vi "Validate message.vi"(0 "multipart message in":string[](array[string]), 11 "error in (no error)":errorcluster) -> (3 "Command Type":T1=enum."instrument_control", 4 "multipart message out":string[](array[string]), 6 "command out":T2=enum."configure_rf", 10 "Valid message?":bool, 14 "Debug info":string, 15 "error out":errorcluster)   [LabVIEW 2019, in "mmW_commands.lvlib"]
doc: "- Validate received message\no check if ZMQ multipart message has (exactly) 3 string elements -> PASS/FAIL\no IF PASSED:\n\" …\n\" extract command > enum\n\" decide if it's instrument command or environment control command type"
uses:
  mmW_commands.lvlib
  TypeDefs/commands.ctl
  TypeDefs/command_types.ctl
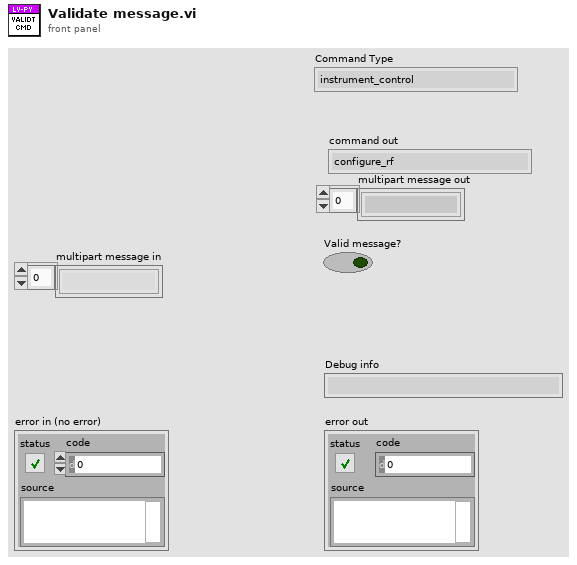
[diagram p1: front panel]
types:
  T1 = typedef "mmW_commands.lvlib/command_types.ctl" = enum16{"invalid_command", "instrument_control", "environment_control", "response"}
  T2 = typedef "mmW_commands.lvlib/commands.ctl" = enum16{"configure_fs", "configure_rf", "configure_trigger", "equalization_enable", "equalization_start", "lo_sync_enable", "equalization_stop", "get_instrument_status", "get_versions", "initialize_hw", "pop_rx", "set_log_level", "Shutdown", "start", "start_instrument_app", "stop", "trans", "transceive", "trigger_burst", "trigger_sync_enable", "Write TX", "resp_generic", "resp_waveform", "send_trigger", "fetch", "transceive2"}
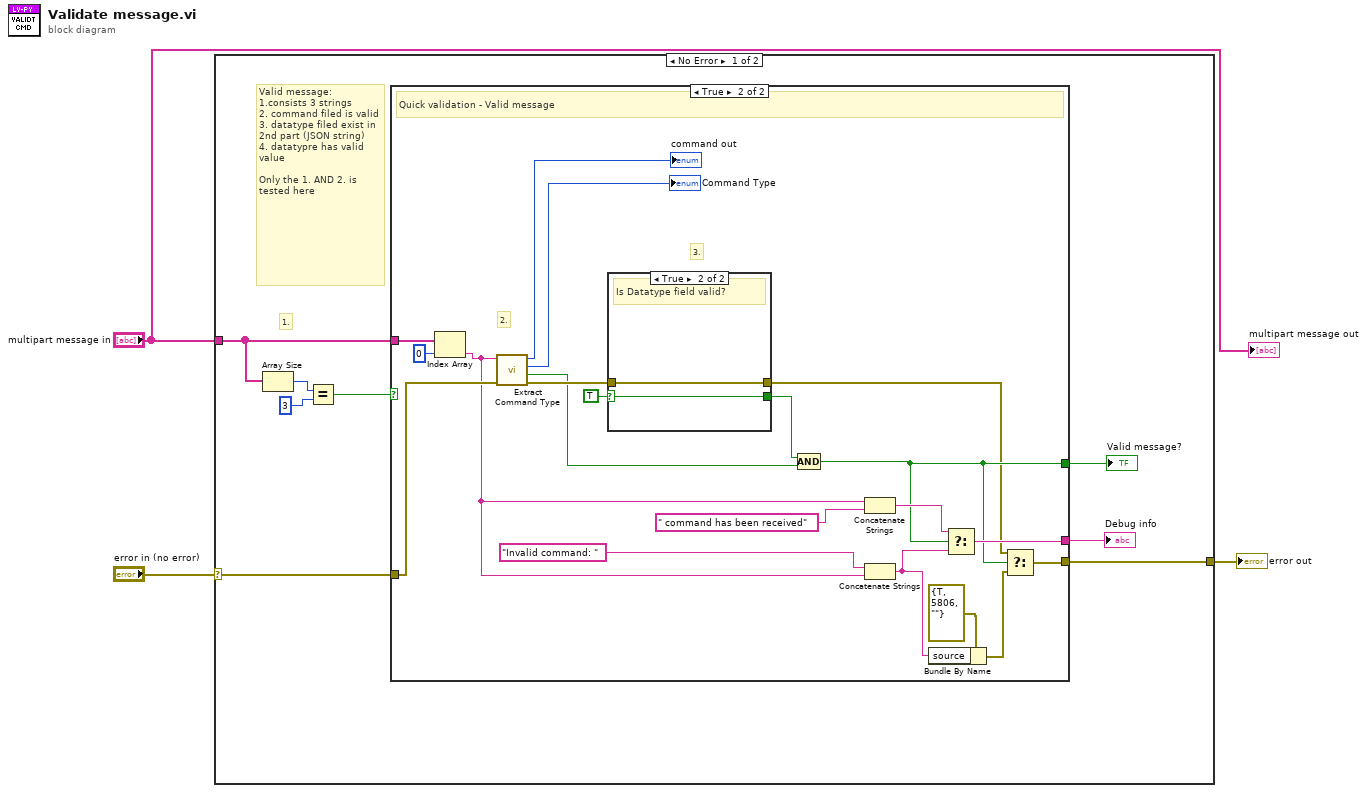
[diagram p0: block diagram]
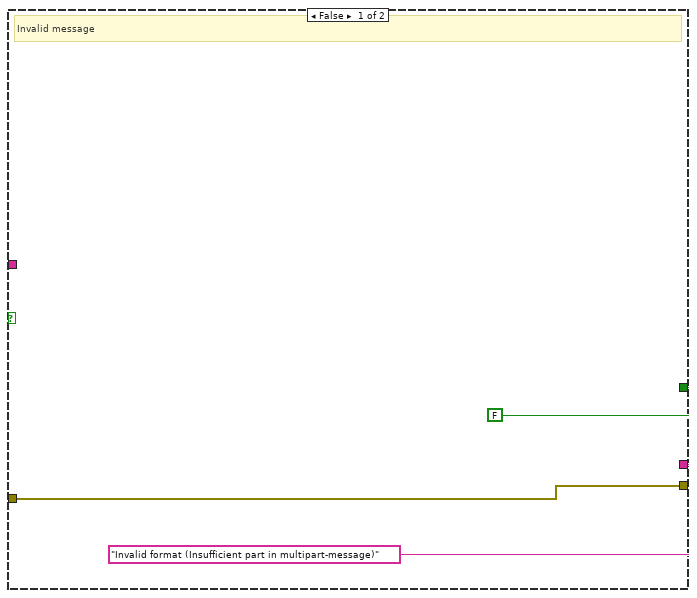
[diagram p2: hidden frame]
diagram:
  n1 = case shown="No Error" "error in (no error)" {
    selector: "error in (no error)" -> [w4 w39]
    tunnel: "multipart message in" -> [w10 _]
    tunnel: [w5 w39] -> w2
    frame No Error {
      # "1."
      # "Valid message:\n1.consists 3 strings\n2. command filed is valid\n3. datatype filed exist in 2nd part (JSON string)\n4. datatypre has valid value\n\nOnly the 1. AND 2. is tested here"
      n2 = Array Size(array=w10) -> (size(s)=w7:i32)
      n3 = Equal?(x=w7, y=3) -> (x = y?=w9:bool)
      n4 = case shown="True" w9 {
        tunnel: w4 -> [w13 w30]
        tunnel: w10 -> [_ w25]
        tunnel: [FALSE w17] -> w6
        tunnel: [w13 w29] -> w5
        tunnel: ["Invalid format (Insufficient part in multipart-message)" w32] -> w11
        frame False {
          # "Invalid message"
        }
        frame True {
          # "3."
          # "2."
          # "Quick validation - Valid message"
          n5 = Index Array(array=w25, index=0) -> (element=w16:string)
          n6 = call "Extract Command Type.vi"("error in (no error)"=w30, "Command field in"=w16) -> ("error out"=w20:errorcluster, "Command valid?"=w18:bool, "Command Type"=→"Command Type":T1, "Command"=→"command out":T2)  [unwired: 5 in, 1 out]
          n7 = case shown="True" TRUE {
            selector: TRUE -> [w35 w37]
            tunnel: w20 -> [w36 w38]
            tunnel: [w36 w38] -> w15
            tunnel: [w35 w37] -> w19
            frame False {
            }
            frame True {
              # "Is Datatype field valid?"
            }
          }
          n8 = Compound Arithmetic op=AND(w19, w18) -> (w17:bool)
          n9 = Concatenate Strings(w16, " command has been received" ("string")) -> (w31:string)
          n10 = Concatenate Strings("Invalid command: " ("f"), w16) -> (w26:string)
          n11 = Bundle By Name(cluster=errorcluster {"status"=TRUE, "code"=5806, "source"=""} ("f"), "source"=w26) -> (w27:errorcluster)
          n12 = Select(t=w31, s=w17, f=w26) -> (s? t:f=w32:string)
          n13 = Select(t=w15, s=w17, f=w27) -> (s? t:f=w29:errorcluster)
        }
      }
      "Debug info" <- w11
      "Valid message?" <- w6
    }
    frame Error {
    }
  }
  "error out" <- w2
  "multipart message out" <- "multipart message in"
